vi "Format Spotlight Text.vi"(6 "Walk":dbl, 9 "A Walk":dbl, 10 "String":string, 11 "String 2":string) -> (3 "String 3":string)   [LabVIEW 2020, in "Visualisation.lvclass"]
uses:
  Visualisation.lvclass
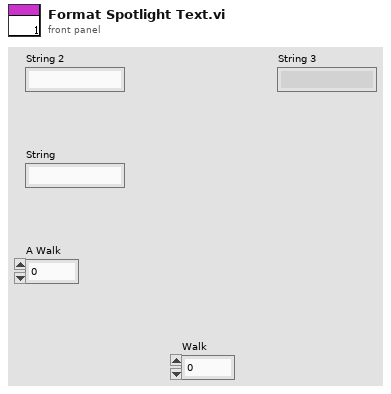
[diagram p1: front panel]
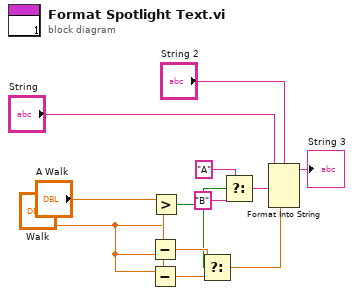
[diagram p0: block diagram]
diagram:
  n1 = Subtract(x="A Walk", y="Walk") -> (x-y=w6:dbl)
  n2 = Subtract(x="Walk", y="A Walk") -> (x-y=w7:dbl)
  n3 = Greater?(x="A Walk", y="Walk") -> (0:w5:bool)
  n4 = Select(t=w6, s=w5, f=w7) -> (s? t:f=w8:dbl)
  n5 = Select(t="A", s=w5, f="B") -> (s? t:f=w11:string)
  n6 = Format Into String(format string="String 2", w11, "String", w8) -> (resulting string=→"String 3":string)  [unwired: 2 in, 1 out]
